vi "Read index_ptr.vi"(8 "error in (no error)":errorcluster, 11 "KD Tree in":refnum<class "KD Tree.lvclass">) -> (0 "error out":errorcluster, 2 "index_ptr":u64, 3 "KD Tree out":refnum<class "KD Tree.lvclass">)   [LabVIEW 2020, in "KD Tree.lvlib" / "KD Tree.lvclass"]
uses:
  KD Tree.lvclass
  KD Tree.lvclass/KD Tree.ctl
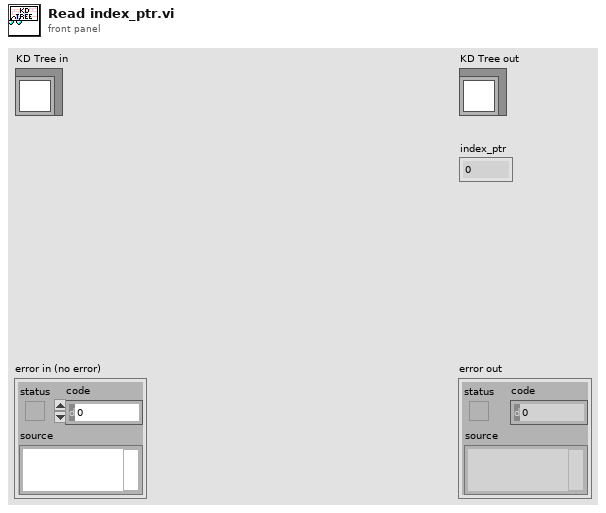
[diagram p1: front panel]
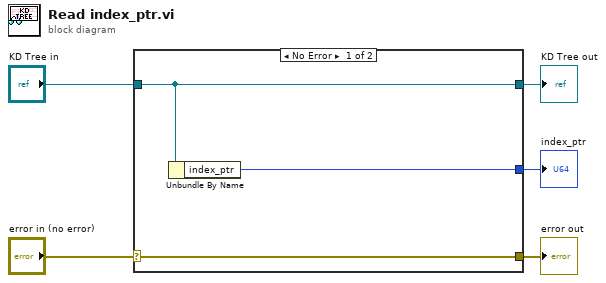
[diagram p0: block diagram]
diagram:
  n1 = case shown="No Error" "error in (no error)" {
    selector: "error in (no error)" -> [w8 w9]
    tunnel: [w8 w9] -> w4
    tunnel: [w7 w10] -> w2
    tunnel: "KD Tree in" -> [w7 w10]
    tunnel: [w6 _] -> w1
    frame No Error {
      n2 = Unbundle By Name(w7) -> ("index_ptr"=w6:u64)
    }
    frame Error {
    }
  }
  "error out" <- w4
  "KD Tree out" <- w2
  "index_ptr" <- w1
